vi "Core Function.vi"() -> ()   [LabVIEW 2020]
uses:
  controls/Core State.ctl
panel:
  in  "Stop":bool
  out "Numeric":i32
  in  "Play":bool
  in  "Media Stop":bool
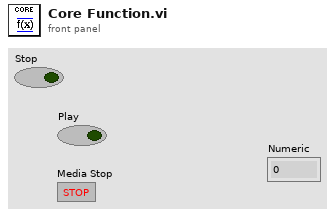
[diagram p1: front panel]
types:
  T1 = typedef "Core State.ctl" = enum16{"Init", "Idle", "Play", "Stop"}
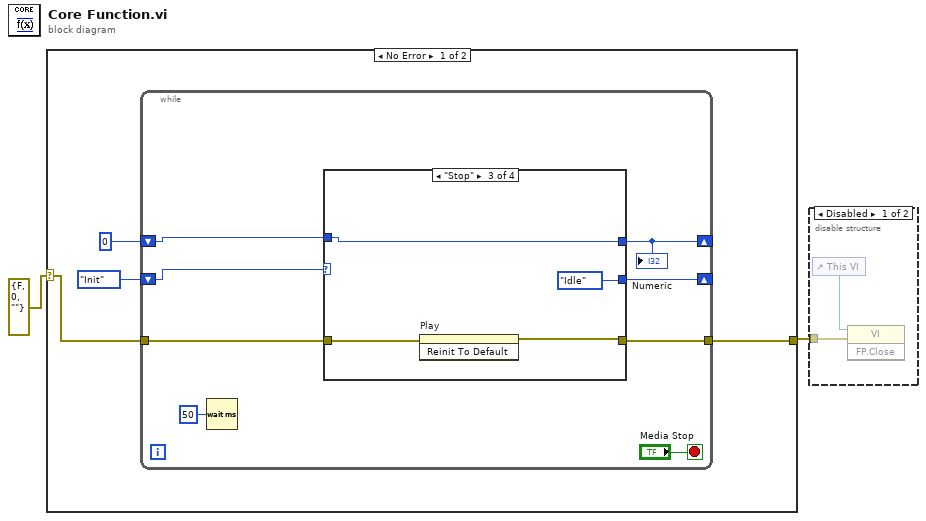
[diagram p0: block diagram]
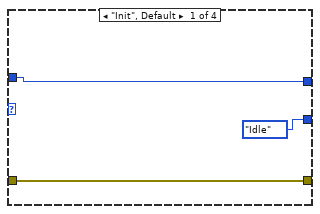
[diagram p3: hidden frame]
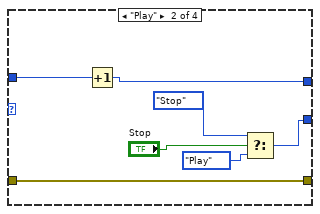
[diagram p4: hidden frame]
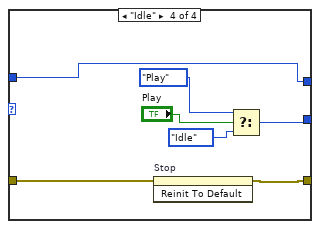
[diagram p5: hidden frame]
diagram:
  n1 = case shown="No Error" errorcluster {"status"=FALSE, "code"=0, "source"=""} ("error constant") {
    selector: errorcluster {"status"=FALSE, "code"=0, "source"=""} ("error constant") -> [w5 w36]
    tunnel: [w4 w36] -> w1
    frame No Error {
      n2 = while {
        shift-right: [w12] -> _
        shift-left: 0 -> [w13]
        tunnel: w5 -> [w10]
        tunnel: [w9] -> w4
        shift-right: [w7] -> _
        shift-left: Core_State."Init" -> [w8]
        stop <- "Media Stop" stop-if-true
        n3 = Wait (ms)(milliseconds to wait=u32 50) -> ()  [unwired: 1 out]
        n4 = case shown="\"Stop\"" w8 {
          tunnel: w13 -> [w17 w24 w28 w31]
          tunnel: [w17 w23 w28 w31] -> w12
          tunnel: w10 -> [w16 w22 w26 w29]
          tunnel: [w16 w22 w25 w30] -> w9
          tunnel: [Core_State."Idle" w19 Core_State."Idle" w35] -> w7
          frame "Init", Default {
          }
          frame "Play" {
            n5 = Increment(x=w24) -> (x+1=w23:i32)
            n6 = Select(t=Core_State."Stop", s="Stop", f=Core_State."Play") -> (s? t:f=w19:T1)
          }
          frame "Stop" {
            n7 = invoke on="Play" class="Bool (strict)" method="Reinit To Default"(error in=w26) -> (error out=w25:errorcluster)  [unwired: 2 in, 2 out]
          }
          frame "Idle" {
            n8 = invoke on="Stop" class="Bool (strict)" method="Reinit To Default"(error in=w29) -> (error out=w30:errorcluster)  [unwired: 2 in, 2 out]
            n9 = Select(t=Core_State."Play", s="Play", f=Core_State."Idle") -> (s? t:f=w35:T1)
          }
        }
        "Numeric" <- w12
      }
    }
    frame Error {
    }
  }
  n10 = disable-structure shown="Disabled" {
    disable-tunnel: w1 -> [w38 _]
    frame Disabled {
      n11 = control-ref of="This VI"() -> (w37:refnum<vi>)
      n12 = invoke class="VI" method="FP.Close"(reference=w37, error in=w38) -> ()  [unwired: 1 in, 3 out]
    }
    frame Enabled {
    }
  }
